vi "WSVCAP SHL Host TL Tester.vi"(0 "FPGA":T1) -> ()   [LabVIEW 2012]
uses:
  Type Defs/WSVCAP SHL DUT Number Enum.ctl
  <vilib>/userdefined/High Color/nirio_resource_hc.ctl
  Type Defs/WSVCAP SHL I2C FPGA Enum.ctl
  Type Defs/WSVCAP SHL Tester System Cluster.ctl
  Type Defs/WSVCAP SHL I2C DUT Mask Mode Enum.ctl
panel:
  in  "C3 Cap DAC":u8=144 caption="B Data In" format="0x%02x"
  in  "C2 Cap DAC":u8=144 caption="B Data In" format="0x%02x"
  in  "C1 Cap DAC":u8=144 caption="B Data In" format="0x%02x"
  in  "Set Cap DAC":bool
  in  "CP 35V":bool
  in  "CP 23.75V":bool
  in  "DVA On":bool
  in  "DVA Off":bool
  in  "CP 44V":bool
  in  "CP 40.25V":bool
  in  "Read Data DUT CMD":string caption="Read Data Out"
  in  "Read DUT":bool
  in  "CP On":bool
  in  "CP Off":bool
  in  "Write DUT":bool
  in  "Write Data DUT":string caption="Write Data Out"
  out "Read Data DUT Out":string caption="Data In"
  in  "Stop RFFE Cycle":bool
  in  "Start RFFE Cycle":bool
  in  "Command":string[](array[string])=["702013B3B3B", "70201000000"]
  in  "Post CMd Delay":dbl[](array[numeric])=[1.2e-05, 5.4e-05] min=0.0 max=0.5 format="%#.0p s"
  in  "Number of Commands":u32=2 min=1 max=4 step=1
  out "Cycle Count":u64=2 min=1 max=4 step=1
  in  "Monitor":bool
  out "AD7747 Values":string[][](table)
  in  "Mode":enum32{"C1", "C2", "C3", "All", "Single"}(radio)
  in  "RFFE Slave Address":u8=144 caption="Slave Address" format="0x%02x"
  out "Activity Log":string
  out "Simulate FPGA":bool
  out "Online":bool
  out "FPGA Resource":T2
  out "Status":string
  out "Busy":bool
  in  "I2C Bytes to Read":u8=1 caption="Bytes" min=1 max=4 step=1
  in  "Device":enum32{"C1", "C2", "C3"}(radio)
  in  "Exit":bool
  out "Read Data I2C":u8[](array[numeric]) caption="Data In" format="0x%02x"
  in  "Read Reg I2C":u8 caption="Register" format="0x%02x"
  in  "Read I2C":bool
  in  "DUT":T3
  in  "Write Data I2C":u8 caption="Data Out" format="0x%02x"
  in  "Write Reg I2C":u8=144 caption="Register" format="0x%02x"
  in  "I2C Init":bool
  in  "Init Data":u8[](array[numeric])=[164, 160, 14, 33] caption="Data Out" format="0x%02x"
  in  "Init Reg":u8[](array[numeric])=[191, 7, 9, 10] caption="Register" format="0x%02x"
  in  "Write I2C":bool
  in  "I2C Slave Address":u8=144 caption="Slave Address" format="0x%02x"
  in  "RFFE Clock Rate (Hz)":dbl=1000000.0 caption="Clock Rate" format="%.1p Hz"
  in  "I2C Clock Rate (Hz)":dbl=100000.0 caption="Clock Rate" format="%.0p Hz"
  in  "Error":errorcluster
  # "WS1050 Tester"
  # "AD7747 (I2C)"
  # "C1"
  # "C2"
  # "C3"
  # "DUT Control (RFFE)"
  # "DUT Cycling (RFFE)"
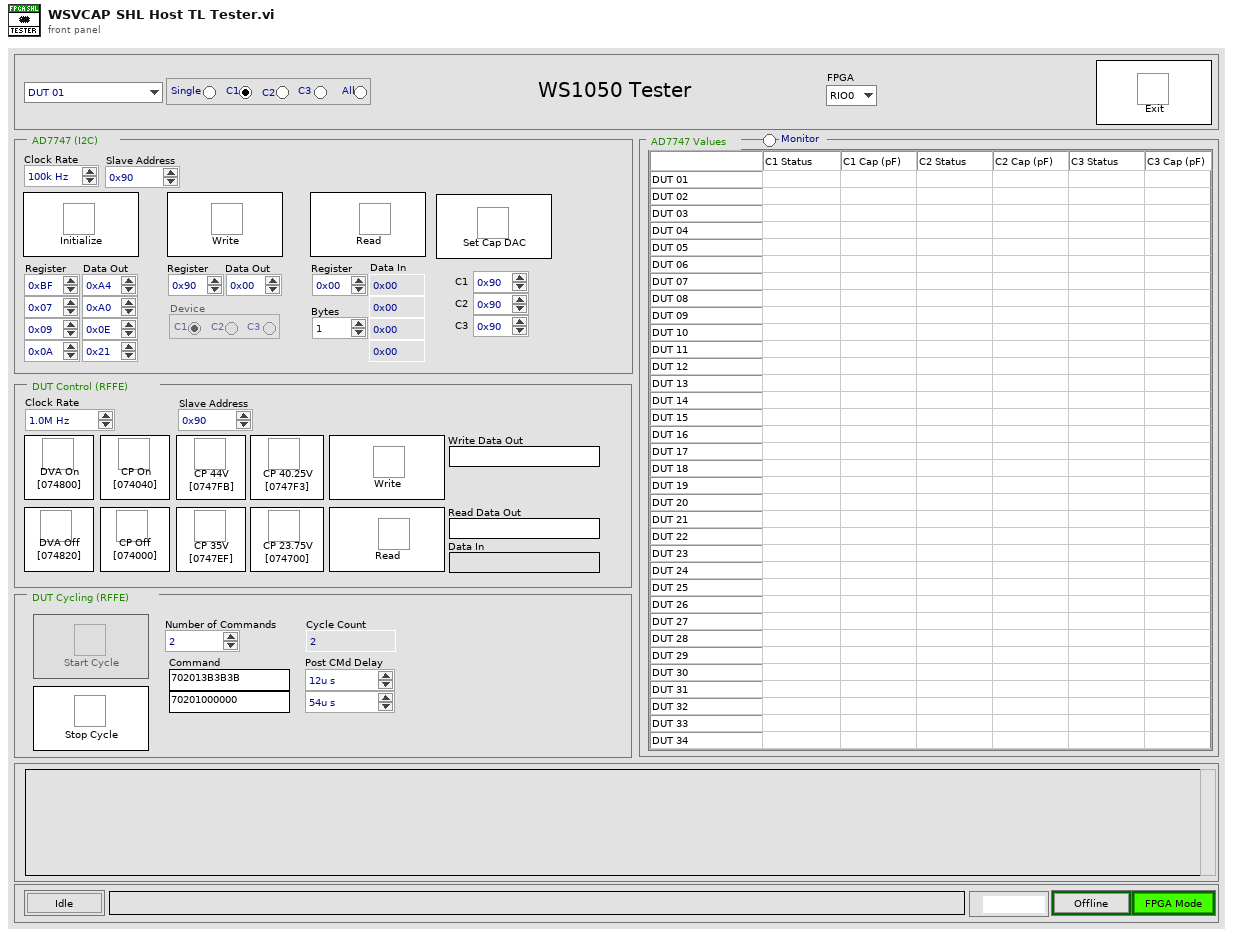
[diagram p1: front panel]
types:
  T1 = typedef "WSVCAP SHL I2C FPGA Enum.ctl" = enum16{"RIO0", "RIO1"}
  T2 = typedef "nirio_resource_hc.ctl" = tag
  T3 = typedef "WSVCAP SHL DUT Number Enum.ctl" = enum16{"DUT 01", "DUT 02", "DUT 03", "DUT 04", "DUT 05", "DUT 06", "DUT 07", "DUT 08", "DUT 09", "DUT 10", "DUT 11", "DUT 12", "DUT 13", "DUT 14", "DUT 15", "DUT 16", "DUT 17", "DUT 18", "DUT 19", "DUT 20", "DUT 21", "DUT 22", "DUT 23", "DUT 24", "DUT 25", "DUT 26", "DUT 27", "DUT 28", "DUT 29", "DUT 30", "DUT 31", "DUT 32", "DUT 33", "DUT 34", "DUT 35", "DUT 36"}
  T4 = typedef "WSVCAP SHL Tester System Cluster.ctl" = cluster{"I2C Monitor":bool, "SPI Cyle":bool, "SPI Mode":enum32{"Write/Read", "Cycle"}, "RFFE Cyle":bool, "RFFE Mode":enum32{"Write/Read", "Cycle"}}
  T5 = typedef "WSVCAP SHL Core System Cluster.ctl" = cluster{"Settings":T6, "FPGA Resource":tag, "Online":bool, "I2C Wait Ticks":u32, "SPI Wait Ticks":u32, "RFFE Wait Ticks":u32, "FPGA VI Reference (FPGA Mode)":T7, "FPGA VI Reference (Sim Mode)":refnum<vi>}
  T6 = typedef "WSVCAP SHL I2C Settings Cluster.ctl" = cluster{"I2C Slave Address":u8, "I2C Clock Rate (Hz)":dbl, "SPI Clock Rate (Hz)":dbl, "RFFE Slave Address":u8, "RFFE Clock Rate (Hz)":dbl, "Simulate FPGA":bool, "C1 Cap DAC Default":u8, "C2 Cap DAC Default":u8, "C3 Cap DAC Default":u8}
  T7 = typedef "WSVCAP SHL FPGA VI Reference.ctl" = refnum<k20>
  T8 = enum8{"Enabled", "Disabled", "Disabled and Grayed Out"}
  T9 = typedef "WSVCAP SHL I2C DUT Mask Mode Enum.ctl" = enum16{"Custom", "C1", "C2", "C3", "All"}
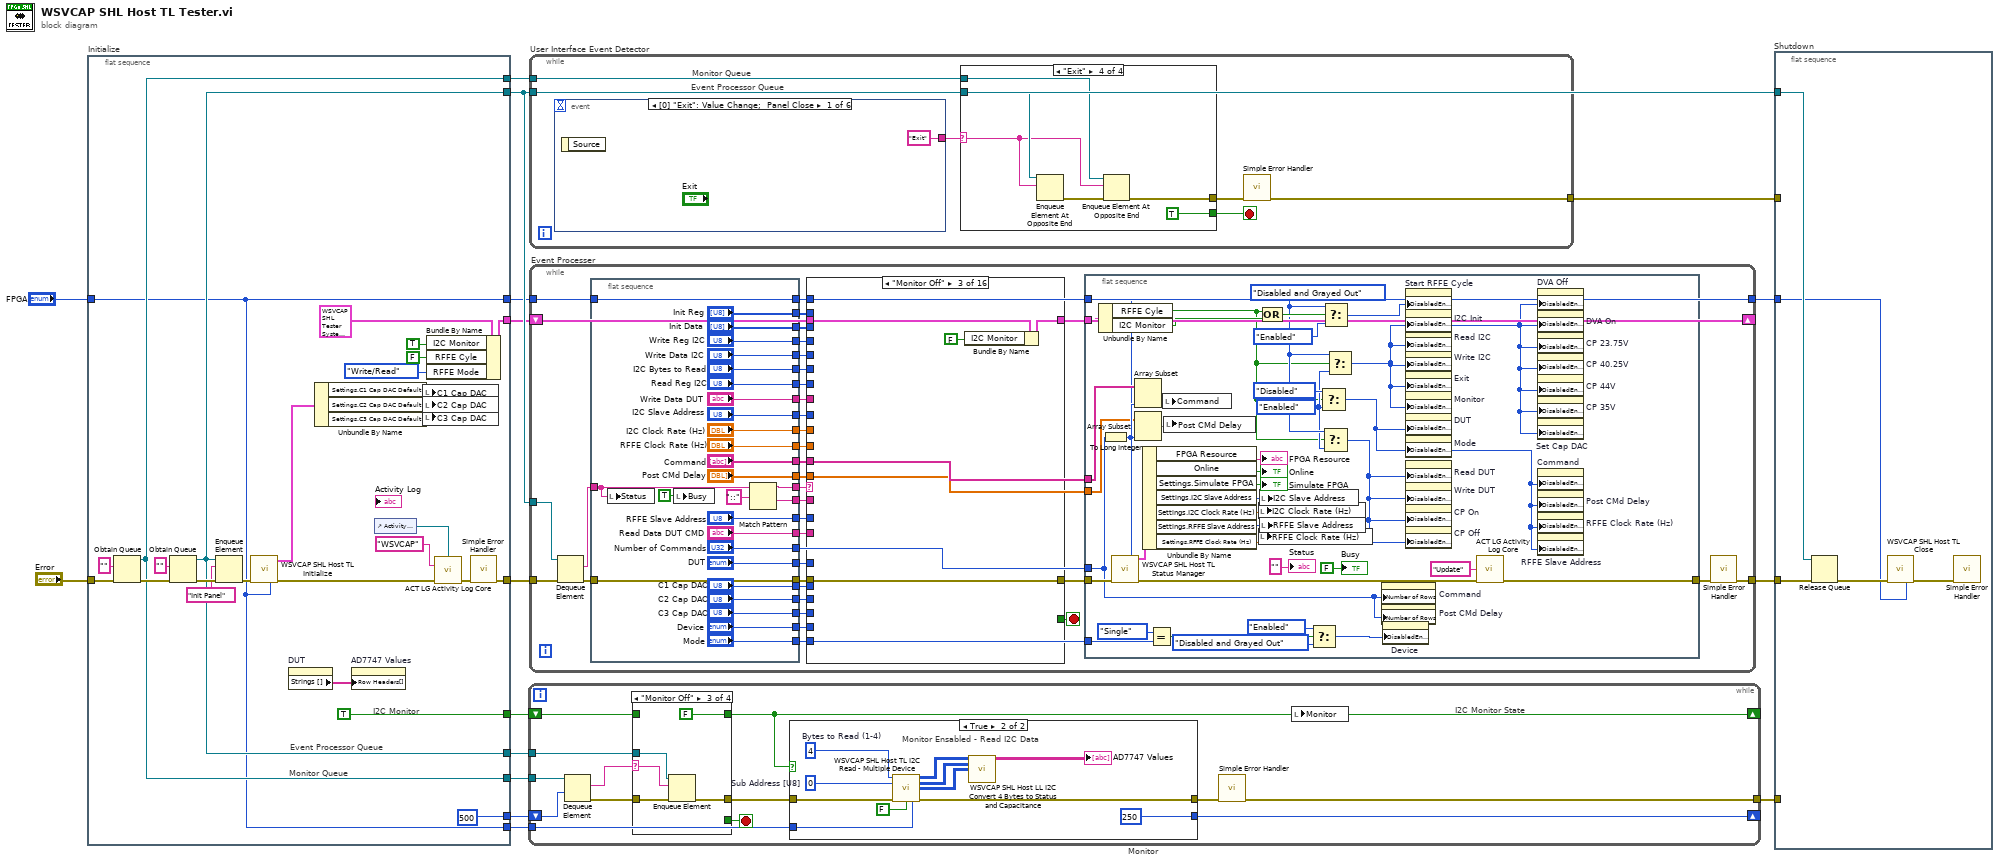
[diagram p0: block diagram]
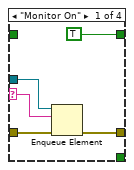
[diagram p2: hidden frame]
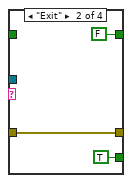
[diagram p3: hidden frame]
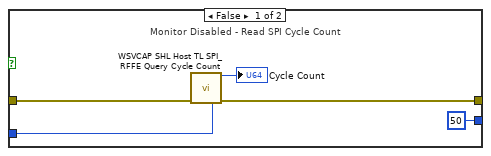
[diagram p5: hidden frame]
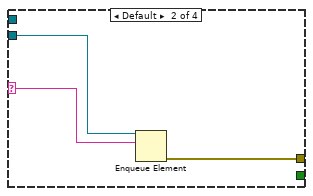
[diagram p7: hidden frame]
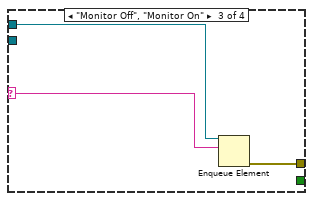
[diagram p8: hidden frame]
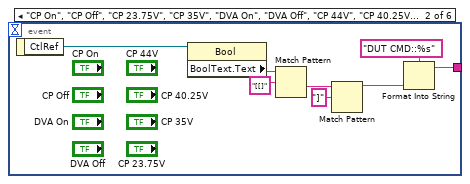
[diagram p9: hidden frame]
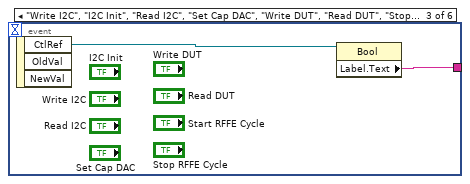
[diagram p10: hidden frame]
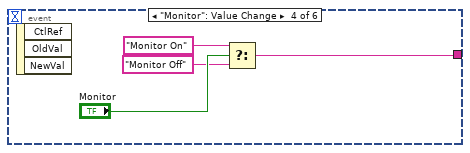
[diagram p11: hidden frame]
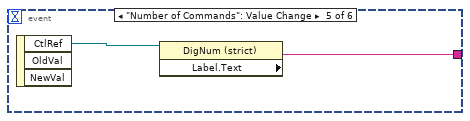
[diagram p12: hidden frame]
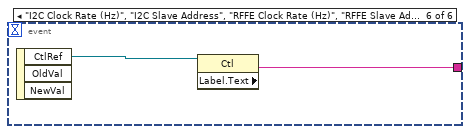
[diagram p13: hidden frame]
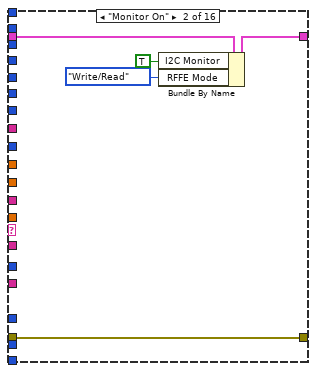
[diagram p15: hidden frame]
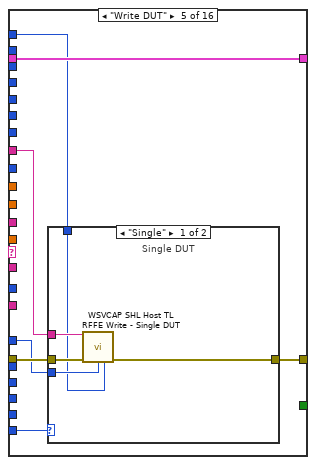
[diagram p17: hidden frame]
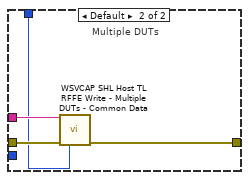
[diagram p18: hidden frame]
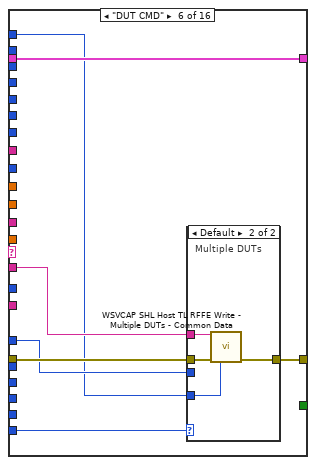
[diagram p19: hidden frame]
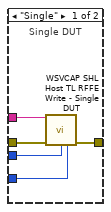
[diagram p20: hidden frame]
diagram:
  n1 = flat-sequence "Initialize" {
    tunnel: "Error" -> [w34]
    tunnel: [w32] -> w15
    tunnel: [TRUE ("Monitor")] -> w6
    tunnel: [w39] -> w11
    tunnel: [w30] -> w10
    tunnel: [w27] -> w9
    tunnel: [w32] -> w8
    tunnel: [w27] -> w7
    tunnel: [500 ("Wait Time (500ms)")] -> w5
    tunnel: "FPGA" -> [w17]
    tunnel: [w17] -> w3
    tunnel: [w17] -> w1
    frame #0 {
      # "I2C Monitor"
      # "Monitor Queue"
      # "Event Processor Queue"
      n2 = Obtain Queue(element data type="" ("name (unnamed)"), error in (no error)=w34) -> (queue out=w27:refnum<queue>, error out=w33:errorcluster)  [unwired: 3 in, 1 out]
      n3 = Obtain Queue(element data type="" ("name (unnamed)"), error in (no error)=w33) -> (queue out=w32:refnum<queue>, error out=w42:errorcluster)  [unwired: 3 in, 1 out]
      n4 = Enqueue Element(queue=w32, element="Init Panel" ("name (unnamed)"), error in (no error)=w42) -> (error out=w24:errorcluster)  [unwired: 1 in, 2 out]
      n5 = call "WSVCAP SHL Host TL Initialize.vi"("error in"=w24, "FPGA"=w17) -> ("System"=w22:T5, "error out"=w23:errorcluster)  [unwired: 12 in]
      n6 = property on="DUT" class="Enum (strict)"() -> ("Strings []"=w25:string[])  [unwired: 2 in, 2 out]
      n7 = Unbundle By Name(w22) -> ("Settings.C1 Cap DAC Default"=w21:u8, "Settings.C2 Cap DAC Default"=w20:u8, "Settings.C3 Cap DAC Default"=w19:u8)
      n8 = property on="AD7747 Values" class="Tbl (strict)"("Row Headers[]"=w25) -> ()  [unwired: 2 in, 2 out]
      n9 = control-ref of="Activity Log"() -> (w38:refnum<vi>)
      n10 = local write "C1 Cap DAC"(w21) -> ()
      n11 = local write "C2 Cap DAC"(w20) -> ()
      n12 = local write "C3 Cap DAC"(w19) -> ()
      n13 = Bundle By Name(cluster=T4 {"I2C Monitor"=TRUE, "SPI Cyle"=TRUE, "SPI Mode"=enum."Write/Read", "RFFE Cyle"=FALSE, "RFFE Mode"=enum."Write/Read"}, "I2C Monitor"=TRUE, "RFFE Cyle"=FALSE ("I2C Monitor"), "RFFE Mode"=enum32{"Write/Read", "Cycle"}."Write/Read" ("SPI Mode")) -> (w30:T4)
      n14 = call "ACT LG Activity Log Core.vi"("Display Ref"=w38, "Source"="WSVCAP", "Error In (no error)"=w23) -> ("Error Out"=w40:errorcluster)  [unwired: 11 in, 1 out]
      n15 = call <vilib>:"Simple Error Handler.vi"("error in (no error)"=w40) -> ("error out"=w39:errorcluster)  [unwired: 4 in, 4 out]
    }
  }
  n16 = while "Monitor" {
    tunnel: [w48] -> w12
    shift-right: [w47] -> _
    shift-left: w6 -> [w54]
    tunnel: w9 -> [w52]
    tunnel: w8 -> [w51]
    shift-right: [w46] -> _
    shift-left: w5 -> [w45]
    tunnel: w1 -> [w44]
    stop <- w49 stop-if-true
    # "I2C Monitor State"
    n17 = Dequeue Element(queue=w52, timeout in ms (-1)=w45) -> (element=w55:string, error out=w53:errorcluster)  [unwired: 1 in, 2 out]
    n18 = case shown="\"Monitor Off\"" w55 {
      selector: w55 -> [w58 _ w66 _]
      tunnel: [TRUE FALSE FALSE w71] -> w47
      tunnel: w54 -> [_ _ _ w71]
      tunnel: w53 -> [w60 w63 w68 w70]
      tunnel: [w59 w63 w67 w70] -> w50
      tunnel: w51 -> [w57 _ w65 _]
      tunnel: [_ TRUE _ _] -> w49
      frame "Monitor On" {
        n19 = Enqueue Element(queue=w57, element=w58, error in (no error)=w60) -> (error out=w59:errorcluster)  [unwired: 1 in, 2 out]
      }
      frame "Exit" {
      }
      frame "Monitor Off" {
        n20 = Enqueue Element(queue=w65, element=w66, error in (no error)=w68) -> (error out=w67:errorcluster)  [unwired: 1 in, 2 out]
      }
      frame Default {
      }
    }
    n21 = case shown="True" w47 {
      tunnel: [w74 w81] -> w56
      tunnel: w50 -> [w75 w82]
      tunnel: [50 ("Wait Time (500ms)") 250 ("Wait Time (500ms)")] -> w46
      tunnel: w44 -> [w72 w77]
      frame False {
        # "Monitor Disabled - Read SPI Cycle Count"
        n22 = call "WSVCAP SHL Host TL SPI_RFFE Query Cycle Count.vi"("error in"=w75, "FPGA"=w72) -> ("Cycle Count"=→"Cycle Count":u64, "error out"=w74:errorcluster)  [unwired: 12 in]
      }
      frame True {
        w86 = u8 4  # Bytes to Read (1-4)
        w87 = u8 0  # Sub Address [U8]
        # "Monitor Ensabled - Read I2C Data"
        n23 = call "WSVCAP SHL Host TL I2C Read - Multiple Device.vi"("Bytes to Read (1-4)"=w86, "Sub Address [U8]"=w87, "error in"=w82, "Log (T)"=FALSE, "FPGA"=w77) -> ("C1:1-36 Read Data [U8]"=w85:u8[][], "C2:1-36 Read Data [U8]"=w84:u8[][], "C3:1-36 Read Data [U8]"=w80:u8[][], "error out"=w81:errorcluster)  [unwired: 7 in]
        n24 = call "WSVCAP SHL Host LL I2C Convert 4 Bytes to Status and Capacitance.vi"("C1:1-36 Read Data [U8]"=w85, "C2_1-36 Read Data [U8]"=w84, "C3_1-36 Read Data [U8]"=w80) -> ("AD7747 Values"=→"AD7747 Values":string[][])  [unwired: 12 in]
      }
    }
    n25 = call <vilib>:"Simple Error Handler.vi"("error in (no error)"=w56) -> ("error out"=w48:errorcluster)  [unwired: 4 in, 4 out]
    n26 = local write "Monitor"(w47) -> ()
  }
  n27 = while "User Interface Event Detector" {
    tunnel: w15 -> [w92]
    tunnel: [w89] -> w13
    tunnel: w7 -> [w88]
    stop <- w90 stop-if-true
    # "Monitor Queue"
    # "Event Processor Queue"
    n28 = event shown="[0] \"Exit\": Value Change;  Panel Close" {
      selector: _ -> [_ _ _ _ _ _]
      dyn-events: _ -> [_ _ _ _ _ _]
      timeout: _ -> [_ _ _ _ _ _]
      tunnel: ["Exit" ("Label.Text") w113 w116 w117 w122 w124] -> w93
      event "Exit": Value Change; Panel Close {
        n29 = event-data() -> ()  [unwired: 1 in, 1 out]
      }
      event "CP On", "CP Off", "CP 23.75V", "CP 35V", "DVA On", "DVA Off", "CP 44V", "CP 40.25V": Value Change {
        n30 = event-data() -> ("CtlRef"=w114:refnum<vi>)  [unwired: 1 in]
        n31 = property class="Bool"(reference=w114) -> ("BoolText.Text"=w111:string)  [unwired: 1 in, 2 out]
        n32 = Match Pattern(string=w111, regular expression="[[]") -> (after substring=w109:string)  [unwired: 1 in, 3 out]
        n33 = Match Pattern(string=w109, regular expression="]") -> (before substring=w107:string)  [unwired: 1 in, 3 out]
        n34 = Format Into String(format string="DUT CMD::%s", w107) -> (resulting string=w113:string)  [unwired: 2 in, 1 out]
      }
      event "Write I2C", "I2C Init", "Read I2C", "Set Cap DAC", "Write DUT", "Read DUT", "Stop RFFE Cycle", "Start RFFE Cycle": Value Change {
        n35 = event-data() -> ("CtlRef"=w115:refnum<vi>)  [unwired: 1 in, 2 out]
        n36 = property class="Bool"(reference=w115) -> ("Label.Text"=w116:string)  [unwired: 1 in, 2 out]
      }
      event "Monitor": Value Change {
        n37 = event-data() -> ()  [unwired: 1 in, 3 out]
        n38 = Select(t="Monitor On" ("Label.Text"), s="Monitor", f="Monitor Off" ("Label.Text")) -> (s? t:f=w117:string)
      }
      event "Number of Commands": Value Change {
        n39 = event-data() -> ("CtlRef"=w121:refnum<vi>)  [unwired: 1 in, 2 out]
        n40 = property class="DigNum (strict)"(reference=w121) -> ("Label.Text"=w122:string)  [unwired: 1 in, 2 out]
      }
      event "I2C Clock Rate (Hz)", "I2C Slave Address", "RFFE Clock Rate (Hz)", "RFFE Slave Address", "Mode": Value Change {
        n41 = event-data() -> ("CtlRef"=w123:refnum<vi>)  [unwired: 1 in, 2 out]
        n42 = property class="Ctl"(reference=w123) -> ("Label.Text"=w124:string)  [unwired: 1 in, 2 out]
      }
    }
    n43 = case shown="\"Exit\"" w93 {
      selector: w93 -> [_ w96 w99 w100]
      tunnel: w92 -> [_ w95 _ w105]
      tunnel: [_ w94 w98 w102] -> w91
      tunnel: [_ _ _ TRUE] -> w90
      tunnel: w88 -> [_ _ w97 w101]
      frame "" {
      }
      frame Default {
        n44 = Enqueue Element(queue=w95, element=w96) -> (error out=w94:errorcluster)  [unwired: 2 in, 2 out]
      }
      frame "Monitor Off", "Monitor On" {
        n45 = Enqueue Element(queue=w97, element=w99) -> (error out=w98:errorcluster)  [unwired: 2 in, 2 out]
      }
      frame "Exit" {
        n46 = Enqueue Element At Opposite End(queue=w105, element=w100) -> (error out=w103:errorcluster)  [unwired: 2 in, 2 out]
        n47 = Enqueue Element At Opposite End(queue=w101, element=w100, error in (no error)=w103) -> (error out=w102:errorcluster)  [unwired: 1 in, 2 out]
      }
    }
    n48 = call <vilib>:"Simple Error Handler.vi"("error in (no error)"=w91) -> ("error out"=w89:errorcluster)  [unwired: 4 in, 4 out]
  }
  n49 = while "Event Processer" {
    tunnel: w15 -> [w160]
    tunnel: [w158] -> w14
    tunnel: w11 -> [w139]
    shift-right: [w134] -> _
    shift-left: w10 -> [w135]
    tunnel: w3 -> [w125]
    tunnel: [w125] -> w2
    stop <- w159 stop-if-true
    n50 = Dequeue Element(queue=w160, error in (no error)=w139) -> (element=w156:string, error out=w154:errorcluster)  [unwired: 1 in, 2 out]
    n51 = flat-sequence {
      tunnel: ["I2C Clock Rate (Hz)"] -> w157
      tunnel: [w206] -> w155
      tunnel: w156 -> [w207]
      tunnel: [w226] -> w153
      tunnel: w154 -> [w226]
      tunnel: ["I2C Bytes to Read"] -> w152
      tunnel: ["I2C Slave Address"] -> w151
      tunnel: ["RFFE Clock Rate (Hz)"] -> w150
      tunnel: ["DUT"] -> w147
      tunnel: ["Init Data"] -> w146
      tunnel: ["Init Reg"] -> w145
      tunnel: ["Write Reg I2C"] -> w144
      tunnel: ["Write Data I2C"] -> w143
      tunnel: ["Read Reg I2C"] -> w142
      tunnel: ["Write Data DUT"] -> w141
      tunnel: ["Mode"] -> w131
      tunnel: ["Device"] -> w140
      tunnel: ["Command"] -> w137
      tunnel: ["Post CMd Delay"] -> w136
      tunnel: ["Number of Commands"] -> w138
      tunnel: ["RFFE Slave Address"] -> w133
      tunnel: ["Read Data DUT CMD"] -> w132
      tunnel: [w204] -> w130
      tunnel: ["C1 Cap DAC"] -> w129
      tunnel: ["C2 Cap DAC"] -> w128
      tunnel: ["C3 Cap DAC"] -> w127
      tunnel: [w200] -> w126
      tunnel: w125 -> [w200]
      frame #0 {
        n52 = local write "Status"(w207) -> ()
        n53 = local write "Busy"(TRUE ("Busy")) -> ()
        n54 = Match Pattern(string=w207, regular expression="::") -> (before substring=w206:string, after substring=w204:string)  [unwired: 1 in, 2 out]
      }
    }
    n55 = case shown="\"Monitor Off\"" w155 {
      tunnel: w153 -> [w229 w234 w238 w240 w247 w263 w279 w306 w323 w332 w354 w369 w402 w404 w411 w417]
      tunnel: [w229 w234 w238 w240 w246 w262 w278 w305 w322 w331 w353 w368 w396 w404 w408 w415] -> w149
      tunnel: [_ _ _ _ _ _ _ _ _ _ _ _ _ TRUE _ _] -> w159
      tunnel: w157 -> [_ _ _ _ _ _ _ _ _ _ _ _ _ _ w410 _]
      tunnel: w152 -> [_ _ _ _ _ _ _ _ _ _ _ _ w398 _ _ _]
      tunnel: w151 -> [_ _ _ _ _ _ _ _ _ _ _ _ _ _ w409 _]
      tunnel: w150 -> [_ _ _ _ _ _ _ _ _ _ _ _ _ _ _ w416]
      tunnel: w147 -> [_ _ _ _ w244 w260 w276 w303 _ w329 _ w366 w401 _ _ _]
      tunnel: w146 -> [_ _ _ _ _ _ _ _ _ _ _ w363 _ _ _ _]
      tunnel: w145 -> [_ _ _ _ _ _ _ _ _ _ _ w364 _ _ _ _]
      tunnel: w144 -> [_ _ _ _ _ _ _ _ _ w327 _ _ _ _ _ _]
      tunnel: w143 -> [_ _ _ _ _ _ _ _ _ w326 _ _ _ _ _ _]
      tunnel: w142 -> [_ _ _ _ _ _ _ _ _ _ _ _ w399 _ _ _]
      tunnel: w141 -> [_ _ _ _ w243 _ _ _ _ _ _ _ _ _ _ _]
      tunnel: w131 -> [_ _ _ _ w245 w261 w277 w304 _ w330 _ w367 _ _ _ _]
      tunnel: w140 -> [_ _ _ _ _ _ _ _ _ w328 _ w365 w400 _ _ _]
      tunnel: w137 -> [_ _ _ _ _ _ _ w302 _ _ _ _ _ _ _ _]
      tunnel: w136 -> [_ _ _ _ _ _ _ w301 _ _ _ _ _ _ _ _]
      tunnel: [w228 w232 w236 w239 w242 w259 w275 w299 w319 w325 w360 w362 w395 w403 w407 w414] -> w134
      tunnel: w135 -> [w228 w233 w237 w239 w242 w259 w275 w300 w320 w325 w360 w362 w395 w403 w407 w414]
      tunnel: w133 -> [_ _ _ _ _ _ _ _ _ _ _ _ _ _ _ w413]
      tunnel: w132 -> [_ _ _ _ _ _ w274 _ _ _ _ _ _ _ _ _]
      tunnel: w130 -> [_ _ _ _ _ w258 _ _ _ _ _ _ _ _ _ _]
      tunnel: w129 -> [_ _ _ _ _ _ _ w297 _ _ w352 _ _ _ _ _]
      tunnel: w128 -> [_ _ _ _ _ _ _ w296 _ _ w351 _ _ _ _ _]
      tunnel: w127 -> [_ _ _ _ _ _ _ w295 _ _ w350 _ _ _ _ _]
      tunnel: w126 -> [_ _ _ _ w241 w257 w273 w294 w318 w324 w349 w361 w394 _ w406 w412]
      frame Default {
      }
      frame "Monitor On" {
        n56 = Bundle By Name(cluster=w233, "I2C Monitor"=TRUE, "RFFE Mode"=enum32{"Write/Read", "Cycle"}."Write/Read" ("SPI Mode")) -> (w232:T4)
      }
      frame "Monitor Off" {
        n57 = Bundle By Name(cluster=w237, "I2C Monitor"=FALSE) -> (w236:T4)
      }
      frame "Number of Commands" {
      }
      frame "Write DUT" {
        n58 = case shown="\"Single\"" w245 {
          tunnel: w247 -> [w252 w256]
          tunnel: [w249 w255] -> w246
          tunnel: w244 -> [w250 _]
          tunnel: w243 -> [w251 w254]
          tunnel: w241 -> [w248 w253]
          frame "Single" {
            # "Single DUT"
            n59 = call "WSVCAP SHL Host TL RFFE Write - Single DUT.vi"("Data Out"=w251, "error in"=w252, "DUT"=w250, "FPGA"=w248) -> ("error out"=w249:errorcluster)  [unwired: 11 in]
          }
          frame Default {
            # "Multiple DUTs"
            n60 = call "WSVCAP SHL Host TL RFFE Write - Multiple DUTs - Common Data.vi"("Data Out"=w254, "error in"=w256, "FPGA"=w253) -> ("error out"=w255:errorcluster)  [unwired: 12 in]
          }
        }
      }
      frame "DUT CMD" {
        n61 = case shown="Default" w261 {
          tunnel: w263 -> [w268 w272]
          tunnel: [w265 w271] -> w262
          tunnel: w260 -> [w266 _]
          tunnel: w258 -> [w267 w270]
          tunnel: w257 -> [w264 w269]
          frame "Single" {
            # "Single DUT"
            n62 = call "WSVCAP SHL Host TL RFFE Write - Single DUT.vi"("Data Out"=w267, "error in"=w268, "DUT"=w266, "FPGA"=w264) -> ("error out"=w265:errorcluster)  [unwired: 11 in]
          }
          frame Default {
            # "Multiple DUTs"
            n63 = call "WSVCAP SHL Host TL RFFE Write - Multiple DUTs - Common Data.vi"("Data Out"=w270, "error in"=w272, "FPGA"=w269) -> ("error out"=w271:errorcluster)  [unwired: 12 in]
          }
        }
      }
      frame "Read DUT" {
        n64 = case shown="Default" w277 {
          tunnel: w279 -> [w285 w293]
          tunnel: [w283 w292] -> w278
          tunnel: w276 -> [w284 w289]
          tunnel: w274 -> [w281 w291]
          tunnel: w273 -> [w280 w286]
          frame "Single" {
            # "Single DUT"
            n65 = call "WSVCAP SHL Host TL RFFE Read - Single DUT.vi"("Data Out"=w281, "error in"=w285, "DUT"=w284, "FPGA"=w280) -> ("Data In"=→"Read Data DUT Out":string, "error out"=w283:errorcluster)  [unwired: 10 in]
          }
          frame Default {
            # "Multiple DUTs"
            n66 = To Long Integer(number=w289) -> (32bit integer=w288:i32)
            n67 = call "WSVCAP SHL Host TL RFFE Read - Multiple DUTs - Common Data.vi"("Data Out"=w291, "error in"=w293, "FPGA"=w286) -> ("RFFE Data In"=w290:string[], "error out"=w292:errorcluster)  [unwired: 11 in]
            n68 = Index Array(array=w290, index=w288) -> (element=w287:string)
            n69 = local write "Read Data DUT Out"(w287) -> ()
          }
        }
      }
      frame "Start RFFE Cycle" {
        n70 = case shown="\"All\"" w304 {
          tunnel: w306 -> [w312 w317]
          tunnel: [w311 w316] -> w305
          tunnel: w303 -> [w310 _]
          tunnel: w302 -> [w309 w315]
          tunnel: w301 -> [w308 w314]
          tunnel: w297 -> [_ _]
          tunnel: w296 -> [_ _]
          tunnel: w295 -> [_ _]
          tunnel: w294 -> [w307 w313]
          frame Default {
            # "Single DUT"
            n71 = call "WSVCAP SHL Host TL RFFE Write Cycle - Single DUT.vi"("Data Out (Cycle Commands)"=w309, "Post Command Delay"=w308, "error in"=w312, "DUT"=w310, "FPGA"=w307) -> ("error out"=w311:errorcluster)  [unwired: 10 in]
          }
          frame "All" {
            # "Multiple DUTs"
            n72 = call "WSVCAP SHL Host TL RFFE Write Cycle - Multiple DUTs - Common Data.vi"("Data Out (Cycle Commands)"=w315, "Post Command Delay"=w314, "error in"=w317, "FPGA"=w313) -> ("error out"=w316:errorcluster)  [unwired: 11 in]
          }
        }
        n73 = Bundle By Name(cluster=w300, "RFFE Cyle"=TRUE ("SPI Cyle")) -> (w299:T4)
      }
      frame "Stop RFFE Cycle" {
        n74 = call "WSVCAP SHL Host TL RFFE Stop Write Cycle.vi"("error in"=w323, "FPGA"=w318) -> ("error out"=w322:errorcluster)  [unwired: 13 in]
        n75 = Bundle By Name(cluster=w320, "RFFE Cyle"=FALSE ("SPI Cyle")) -> (w319:T4)
      }
      frame "Write I2C" {
        n76 = case shown="Default" w330 {
          selector: w330 -> [_ w344]
          tunnel: w332 -> [w339 w348]
          tunnel: [w338 w347] -> w331
          tunnel: w329 -> [w336 _]
          tunnel: w327 -> [w335 w346]
          tunnel: w328 -> [w337 _]
          tunnel: w326 -> [w334 w345]
          tunnel: w324 -> [w333 w340]
          frame "Single" {
            # "Single DUT"
            n77 = call "WSVCAP SHL Host TL I2C Write - Single Device.vi"("Sub Address [U8]"=w335, "FPGA"=w333, "Data Out [U8]"=w334, "error in"=w339, "DUT"=w336, "Device"=w337) -> ("error out"=w338:errorcluster)  [unwired: 9 in]
          }
          frame Default {
            # "Multiple DUTs"
            n78 = Format Into String(w344) -> (resulting string=w343:string)  [unwired: 3 in, 1 out]
            n79 = Scan From String(input string=w343, default 1=WSVCAP_SHL_I2C_DUT_Mask_Mode_Enum."All" ("DUT Mask Mode (All)")) -> (output 1=w341:T9)  [unwired: 3 in, 3 out]
            n80 = call "WSVCAP SHL Host TL I2C Write - Multiple Device - Common Data.vi"("Sub Address"=w346, "FPGA"=w340, "Data Out [U8]"=w345, "error in"=w348, "DUT Mask Mode (All)"=w341) -> ("error out"=w347:errorcluster)  [unwired: 10 in]
          }
        }
      }
      frame "Set Cap DAC" {
        w359 = 36 ("dimension size")
        n81 = Initialize Array(w352, w359) -> (w358:u8[])
        n82 = Initialize Array(w351, w359) -> (w357:u8[])
        n83 = Initialize Array(w350, w359) -> (w356:u8[])
        n84 = call "WSVCAP SHL Host TL I2C Write - Multiple Device - Unique Data.vi"("C1 Data"=w358, "FPGA"=w349, "C2 Data"=w357, "C3 Data"=w356, "Sub Address"=u8 11, "error in"=w354) -> ("error out"=w353:errorcluster)  [unwired: 9 in]
      }
      frame "I2C Init" {
        n85 = for {
          tunnel: w367 -> [w375]
          tunnel: w366 -> [w374]
          tunnel: w365 -> [w373]
          tunnel: w364 -> [w372] mode=indexing
          tunnel: w363 -> [w371] mode=indexing
          shift-right: [w376] -> w368
          shift-left: w369 -> [w377]
          tunnel: w361 -> [w370]
          n86 = case shown="Default" w375 {
            selector: w375 -> [_ w387]
            tunnel: w377 -> [w384 w393]
            tunnel: [w383 w392] -> w376
            tunnel: w374 -> [w381 _]
            tunnel: w373 -> [w382 _]
            tunnel: w372 -> [w380 w391]
            tunnel: w371 -> [w379 w390]
            tunnel: w370 -> [w378 w385]
            frame "Single" {
              # "Single DUT"
              n87 = call "WSVCAP SHL Host TL I2C Write - Single Device.vi"("Sub Address [U8]"=w380, "FPGA"=w378, "Data Out [U8]"=w379, "error in"=w384, "DUT"=w381, "Device"=w382) -> ("error out"=w383:errorcluster)  [unwired: 9 in]
            }
            frame Default {
              # "Multiple DUTs"
              n88 = Format Into String(w387) -> (resulting string=w389:string)  [unwired: 3 in, 1 out]
              n89 = Scan From String(input string=w389, default 1=WSVCAP_SHL_I2C_DUT_Mask_Mode_Enum."All" ("DUT Mask Mode (All)")) -> (output 1=w386:T9)  [unwired: 3 in, 3 out]
              n90 = call "WSVCAP SHL Host TL I2C Write - Multiple Device - Common Data.vi"("Sub Address"=w391, "FPGA"=w385, "Data Out [U8]"=w390, "error in"=w393, "DUT Mask Mode (All)"=w386) -> ("error out"=w392:errorcluster)  [unwired: 10 in]
            }
          }
        }
      }
      frame "Read I2C" {
        n91 = call "WSVCAP SHL Host TL I2C Read - Single Device.vi"("Bytes to Read (1-4)"=w398, "FPGA"=w394, "Sub Address [U8]"=w399, "error in"=w402, "DUT"=w401, "Device"=w400) -> ("Device Data"=→"Read Data I2C":u8[], "error out"=w396:errorcluster)  [unwired: 8 in]
      }
      frame "Exit" {
      }
      frame "I2C Clock Rate (Hz)", "I2C Slave Address" {
        n92 = call "WSVCAP SHL Host TL I2C Configure.vi"("I2C_Slave Address"=w409, "Clock Rate (Hz)"=w410, "error in"=w411, "FPGA"=w406) -> ("error out"=w408:errorcluster)  [unwired: 10 in, 1 out]
      }
      frame "RFFE Clock Rate (Hz)", "RFFE Slave Address" {
        n93 = call "WSVCAP SHL Host TL RFFE Configure.vi"("RFFE Slave Address"=w413, "Clock Rate (Hz)"=w416, "error in"=w417, "FPGA"=w412) -> ("error out"=w415:errorcluster)  [unwired: 10 in, 1 out]
      }
    }
    n94 = flat-sequence {
      tunnel: [w187] -> w148
      tunnel: w149 -> [w197]
      tunnel: w138 -> [w186]
      tunnel: w137 -> [w184]
      tunnel: w136 -> [w182]
      tunnel: w134 -> [w180]
      tunnel: w131 -> [w170]
      tunnel: w125 -> [w161]
      frame #0 {
        w174 = T8."Enabled" ("Disabled")
        w175 = T8."Disabled and Grayed Out" ("Disabled")
        n95 = Unbundle By Name(w180) -> ("RFFE Cyle"=w173:bool, "I2C Monitor"=w179:bool)
        n96 = To Long Integer(number=w186) -> (32bit integer=w185:i32)
        n97 = call "WSVCAP SHL Host TL Status Manager.vi"("error in"=w197, "FPGA"=w161) -> ("System Out"=w196:T5, "error out"=w189:errorcluster)  [unwired: 12 in]
        n98 = Array Subset(array=w184, length=w185) -> (w183:string[])  [unwired: 1 in]
        n99 = Array Subset(array=w182, length=w185) -> (w181:dbl[])  [unwired: 1 in]
        n100 = Unbundle By Name(w196) -> ("FPGA Resource"=→"FPGA Resource":tag, "Online"=→"Online":bool, "Settings.Simulate FPGA"=→"Simulate FPGA":bool, "Settings.I2C Slave Address"=w195:u8, "Settings.I2C Clock Rate (Hz)"=w194:dbl, "Settings.RFFE Slave Address"=w171:u8, "Settings.RFFE Clock Rate (Hz)"=w193:dbl)
        n101 = Equal?(x=enum32{"C1", "C2", "C3", "All", "Single"}."Single" ("Mode"), y=w170) -> (x = y?=w166:bool)
        n102 = local write "Command"(w183) -> ()
        n103 = local write "Post CMd Delay"(w181) -> ()
        n104 = local write "I2C Clock Rate (Hz)"(w194) -> ()
        n105 = local write "RFFE Clock Rate (Hz)"(w193) -> ()
        n106 = local write "I2C Slave Address"(w195) -> ()
        n107 = local write "RFFE Slave Address"(w171) -> ()
        n108 = Compound Arithmetic op=OR(w173, w179) -> (w176:bool)
        n109 = Select(t=T8."Enabled" ("Disabled"), s=w166, f=T8."Disabled and Grayed Out" ("Disabled")) -> (s? t:f=w165:T8)
        n110 = Select(t=T8."Disabled" ("Disabled"), s=w173, f=w174) -> (s? t:f=w164:T8)
        n111 = Select(t=w175, s=w173, f=w174) -> (s? t:f=w162:T8)
        n112 = Select(t=w175, s=w176, f=T8."Enabled" ("Disabled")) -> (s? t:f=w172:T8)
        n113 = Select(t=w175, s=w173, f=w174) -> (s? t:f=w163:T8)
        n114 = property on="Command" class="Arr (strict)"("Number of Rows"=w186) -> ()  [unwired: 2 in, 2 out]
        n115 = property on="Post CMd Delay" class="Arr (strict)"("Number of Rows"=w186) -> ()  [unwired: 2 in, 2 out]
        n116 = property on="Device" class="RadioBtnsControl (strict)"("DisabledEnum"=w165) -> ()  [unwired: 2 in, 2 out]
        n117 = property on="Start RFFE Cycle" class="Bool"("DisabledEnum"=w172) -> ()  [unwired: 2 in, 2 out]
        n118 = property on="I2C Init" class="Bool"("DisabledEnum"=w163) -> ()  [unwired: 2 in, 2 out]
        n119 = property on="Read I2C" class="Bool"("DisabledEnum"=w163) -> ()  [unwired: 2 in, 2 out]
        n120 = property on="Write I2C" class="Bool"("DisabledEnum"=w163) -> ()  [unwired: 2 in, 2 out]
        n121 = property on="Exit" class="Bool"("DisabledEnum"=w163) -> ()  [unwired: 2 in, 2 out]
        n122 = property on="Monitor" class="Bool (strict)"("DisabledEnum"=w163) -> ()  [unwired: 2 in, 2 out]
        n123 = property on="DUT" class="Enum (strict)"("DisabledEnum"=w164) -> ()  [unwired: 2 in, 2 out]
        n124 = property on="Mode" class="RadioBtnsControl (strict)"("DisabledEnum"=w164) -> ()  [unwired: 2 in, 2 out]
        n125 = property on="Read DUT" class="Bool"("DisabledEnum"=w162) -> ()  [unwired: 2 in, 2 out]
        n126 = property on="Write DUT" class="Bool"("DisabledEnum"=w162) -> ()  [unwired: 2 in, 2 out]
        n127 = property on="CP On" class="Bool"("DisabledEnum"=w162) -> ()  [unwired: 2 in, 2 out]
        n128 = property on="CP Off" class="Bool"("DisabledEnum"=w162) -> ()  [unwired: 2 in, 2 out]
        n129 = call "ACT LG Activity Log Core.vi"("Log Line"="Update", "Error In (no error)"=w189) -> ("Error Out"=w187:errorcluster)  [unwired: 12 in, 1 out]
        n130 = property on="DVA Off" class="Bool"("DisabledEnum"=w163) -> ()  [unwired: 2 in, 2 out]
        n131 = property on="DVA On" class="Bool"("DisabledEnum"=w163) -> ()  [unwired: 2 in, 2 out]
        n132 = property on="CP 23.75V" class="Bool"("DisabledEnum"=w163) -> ()  [unwired: 2 in, 2 out]
        n133 = property on="CP 40.25V" class="Bool"("DisabledEnum"=w163) -> ()  [unwired: 2 in, 2 out]
        n134 = property on="CP 44V" class="Bool"("DisabledEnum"=w163) -> ()  [unwired: 2 in, 2 out]
        n135 = property on="CP 35V" class="Bool"("DisabledEnum"=w163) -> ()  [unwired: 2 in, 2 out]
        n136 = property on="Set Cap DAC" class="Bool"("DisabledEnum"=w163) -> ()  [unwired: 2 in, 2 out]
        n137 = property on="Command" class="Arr (strict)"("DisabledEnum"=w164) -> ()  [unwired: 2 in, 2 out]
        n138 = property on="Post CMd Delay" class="Arr (strict)"("DisabledEnum"=w164) -> ()  [unwired: 2 in, 2 out]
        n139 = property on="RFFE Clock Rate (Hz)" class="DigNum (strict)"("DisabledEnum"=w164) -> ()  [unwired: 2 in, 2 out]
        n140 = property on="RFFE Slave Address" class="DigNum (strict)"("DisabledEnum"=w164) -> ()  [unwired: 2 in, 2 out]
        "Busy" <- FALSE ("Busy")
        "Status" <- "" ("Status")
      }
    }
    n141 = call <vilib>:"Simple Error Handler.vi"("error in (no error)"=w148) -> ("error out"=w158:errorcluster)  [unwired: 4 in, 4 out]
  }
  n142 = flat-sequence "Shutdown" {
    tunnel: w15 -> [w422]
    tunnel: w14 -> [w421]
    tunnel: w13 -> [_]
    tunnel: w12 -> [_]
    tunnel: w2 -> [w418]
    frame #0 {
      n143 = Release Queue(queue=w422, error in (no error)=w421) -> (error out=w420:errorcluster)  [unwired: 1 in, 2 out]
      n144 = call "WSVCAP SHL Host TL Close.vi"("error in"=w420, "FPGA"=w418) -> ("error out"=w419:errorcluster)  [unwired: 13 in]
      n145 = call <vilib>:"Simple Error Handler.vi"("error in (no error)"=w419) -> ()  [unwired: 4 in, 5 out]
    }
  }
